vi "Read Inputs.vi"(1 "Slider 2":dbl, 2 "Slider 1":dbl) -> (0 "Inputs":cluster{"Slider 1":dbl, "Slider 2":dbl})   [LabVIEW 2012]
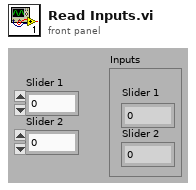
[diagram p1: front panel]
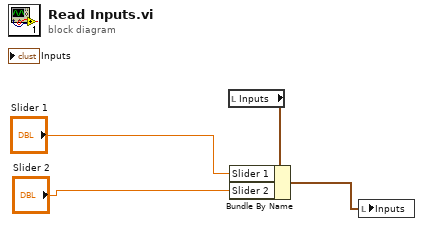
[diagram p0: block diagram]
diagram:
  n1 = local read "Inputs"() -> (w3:cluster{"Slider 1":dbl, "Slider 2":dbl})
  n2 = Bundle By Name(cluster=w3, "Slider 1"="Slider 1", "Slider 2"="Slider 2") -> (w4:cluster{"Slider 1":dbl, "Slider 2":dbl})
  n3 = local write "Inputs"(w4) -> ()
